vi "SR530 read.vi"(11 "SR530":refnum<visa-resource-name>="COM2") -> (3 "Result":string)   [LabVIEW 2015]
panel:
  in  "Write command":string="QX"
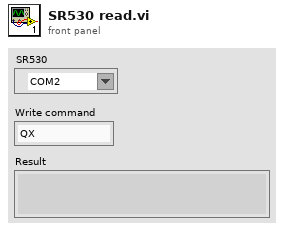
[diagram p1: front panel]
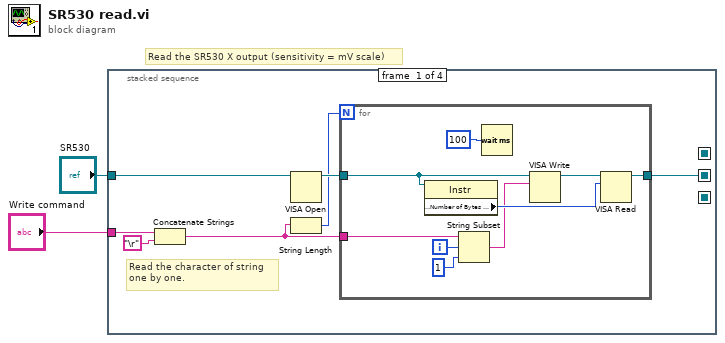
[diagram p0: block diagram]
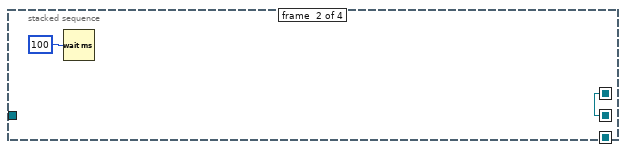
[diagram p2: hidden frame]
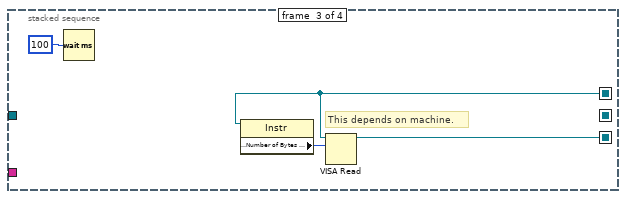
[diagram p3: hidden frame]
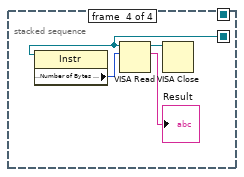
[diagram p4: hidden frame]
diagram:
  # "Read the SR530 X output (sensitivity = mV scale)"
  n1 = stacked-sequence {
    seq-local: [w8 _ _ _] -> [_ w19 _ _]
    seq-local: [_ w19 _ _] -> [_ _ w23 _]
    seq-local: [_ _ w24 _] -> [_ _ _ w27]
    tunnel: "SR530" -> [w5 _ _ _]
    tunnel: "Write command" -> [w4 _ _ _]
    frame #0 {
      # "Read the character of string \none by one."
      n2 = Concatenate Strings(w4, "\r") -> (w7:string)
      n3 = VISA Open(VISA resource name=w5) -> (VISA resource name=w9:refnum<visa-resource-name>)  [unwired: 4 in, 1 out]
      n4 = String Length(string=w7) -> (length=w6:i32)
      n5 = for {
        N: w6 -> [_]
        tunnel: w7 -> [w17]
        tunnel: w9 -> [w16]
        tunnel: [w13] -> w8
        i -> [w15]
        n6 = property class="Instr"(reference=w16) -> ("Serial Settings:Number of Bytes at Serial Port"=w12:u32)  [unwired: 1 in, 2 out]
        n7 = String Subset(string=w17, offset (0)=w15, length (rest)=1 ("length (rest)")) -> (substring=w11:string)
        n8 = Wait (ms)(milliseconds to wait=u32 100) -> ()  [unwired: 1 out]
        n9 = VISA Write(VISA resource name=w16, write buffer=w11) -> (VISA resource name out=w14:refnum<visa-resource-name>)  [unwired: 1 in, 2 out]
        n10 = VISA Read(VISA resource name=w14, byte count=w12) -> (VISA resource name out=w13:refnum<visa-resource-name>)  [unwired: 1 in, 3 out]
      }
    }
    frame #1 {
      n11 = Wait (ms)(milliseconds to wait=u32 100) -> ()  [unwired: 1 out]
    }
    frame #2 {
      # "This depends on machine."
      n12 = Wait (ms)(milliseconds to wait=u32 100) -> ()  [unwired: 1 out]
      n13 = property class="Instr"(reference=w23) -> ("Serial Settings:Number of Bytes at Serial Port"=w22:u32)  [unwired: 1 in, 2 out]
      n14 = VISA Read(VISA resource name=w23, byte count=w22) -> (VISA resource name out=w24:refnum<visa-resource-name>)  [unwired: 1 in, 3 out]
    }
    frame #3 {
      n15 = property class="Instr"(reference=w27) -> ("Serial Settings:Number of Bytes at Serial Port"=w26:u32)  [unwired: 1 in, 2 out]
      n16 = VISA Read(VISA resource name=w27, byte count=w26) -> (VISA resource name out=w25:refnum<visa-resource-name>, read buffer=→"Result":string)  [unwired: 1 in, 2 out]
      n17 = VISA Close(VISA resource name=w25) -> ()  [unwired: 1 in, 1 out]
    }
  }
